vi "HFRR ADV v025 new software.vi"() -> ()   [LabVIEW 2025] (continued)
    shift-left: w3 -> [w1664]
    shift-right: [w1669] -> _
    shift-left: w3 -> [w1663]
    shift-right: [w1668] -> _
    shift-left: w3 -> [w1662]
    shift-right: [w1667] -> _
    shift-left: w3 -> [w1661]
    shift-right: [w1666] -> _
    shift-left: w3 -> [w1660]
    shift-right: [w1665] -> _
    shift-left: w3 -> [w1659]
    shift-right: [w1650] -> _
    shift-left: w3 -> [w1653]
    shift-right: [w1649] -> _
    shift-left: w3 -> [w1652]
    shift-right: [w1648] -> _
    shift-left: w3 -> [w1651]
    stop <- w1698 stop-if-true
    n1472 = local read "Read UNO"() -> (w1657:string)
    n1473 = local read "Error  2"() -> (w1697:errorcluster)
    n1474 = String Length(string=w1657) -> (length=w1656:i32)
    n1475 = call <vilib>:"Trim Whitespace.vi"("string"=w1657) -> ("trimmed string"=w1658:string)  [unwired: 1 in]
    n1476 = Greater Or Equal?(x=w1656, y=23) -> (x >= y?=w1654:bool)
    n1477 = case shown="No Error" w1697 {
      tunnel: w1696 -> [w1744 w1840]
      tunnel: w1695 -> [w1743 w1839]
      tunnel: w1694 -> [w1742 w1838]
      tunnel: w1693 -> [w1741 w1837]
      tunnel: [w1740 w1840] -> w1692
      tunnel: [w1739 w1839] -> w1691
      tunnel: [w1738 w1838] -> w1690
      tunnel: [w1737 w1837] -> w1689
      tunnel: w1688 -> [w1736 w1836]
      tunnel: [w1735 w1836] -> w1687
      tunnel: w1685 -> [w1734 w1835]
      tunnel: w1686 -> [w1733 w1834]
      tunnel: [w1732 w1835] -> w1684
      tunnel: [w1731 w1834] -> w1683
      tunnel: w1682 -> [w1730 w1833]
      tunnel: w1681 -> [w1729 w1832]
      tunnel: w1680 -> [w1728 w1831]
      tunnel: w1679 -> [w1727 w1830]
      tunnel: w1678 -> [w1726 w1829]
      tunnel: w1677 -> [w1725 w1828]
      tunnel: [w1724 w1833] -> w1676
      tunnel: [w1723 w1832] -> w1675
      tunnel: [w1722 w1831] -> w1674
      tunnel: [w1721 w1830] -> w1673
      tunnel: [w1720 w1829] -> w1672
      tunnel: [w1719 w1828] -> w1671
      tunnel: w1664 -> [w1718 w1827]
      tunnel: [w1717 w1827] -> w1670
      tunnel: [w1716 w1823] -> w1669
      tunnel: [w1715 w1822] -> w1668
      tunnel: [w1714 w1826] -> w1667
      tunnel: [w1713 w1825] -> w1666
      tunnel: [w1712 w1824] -> w1665
      tunnel: w1663 -> [w1711 w1826]
      tunnel: w1662 -> [w1710 w1825]
      tunnel: w1661 -> [w1709 w1824]
      tunnel: w1660 -> [w1708 w1823]
      tunnel: w1659 -> [w1707 w1822]
      tunnel: w1658 -> [w1706 _]
      tunnel: w1654 -> [w1705 _]
      tunnel: w1653 -> [w1704 w1821]
      tunnel: w1652 -> [w1703 w1820]
      tunnel: w1651 -> [w1702 w1819]
      tunnel: [w1701 w1821] -> w1650
      tunnel: [w1700 w1820] -> w1649
      tunnel: [w1699 w1819] -> w1648
      frame No Error {
        n1478 = case shown="True" w1705 {
          tunnel: w1744 -> [w1760 w1812]
          tunnel: w1743 -> [w1759 w1811]
          tunnel: w1742 -> [w1758 w1810]
          tunnel: w1741 -> [w1757 w1809]
          tunnel: [w1760 w1808] -> w1740
          tunnel: [w1759 w1807] -> w1739
          tunnel: [w1758 w1806] -> w1738
          tunnel: [w1757 w1805] -> w1737
          tunnel: w1736 -> [w1756 w1803]
          tunnel: [w1756 w1802] -> w1735
          tunnel: w1734 -> [w1755 w1801]
          tunnel: w1733 -> [w1754 w1800]
          tunnel: [w1755 w1799] -> w1732
          tunnel: [w1754 w1798] -> w1731
          tunnel: w1730 -> [w1753 w1797]
          tunnel: w1729 -> [w1752 w1796]
          tunnel: w1728 -> [w1751 w1795]
          tunnel: w1727 -> [w1750 w1794]
          tunnel: w1726 -> [w1749 w1793]
          tunnel: w1725 -> [w1748 w1792]
          tunnel: [w1753 w1791] -> w1724
          tunnel: [w1752 w1790] -> w1723
          tunnel: [w1751 w1789] -> w1722
          tunnel: [w1750 w1788] -> w1721
          tunnel: [w1749 w1787] -> w1720
          tunnel: [w1748 w1786] -> w1719
          tunnel: w1718 -> [w1766 w1785]
          tunnel: [w1766 w1784] -> w1717
          tunnel: [w1763 w1783] -> w1716
          tunnel: [w1762 w1782] -> w1715
          tunnel: [w1765 w1781] -> w1714
          tunnel: [w1761 w1780] -> w1713
          tunnel: [w1764 w1779] -> w1712
          tunnel: w1711 -> [w1765 w1778]
          tunnel: w1710 -> [w1764 w1777]
          tunnel: w1709 -> [w1763 w1776]
          tunnel: w1708 -> [w1762 w1775]
          tunnel: w1707 -> [w1761 w1774]
          tunnel: w1706 -> [_ w1773]
          tunnel: w1704 -> [w1747 w1772]
          tunnel: w1703 -> [w1746 w1771]
          tunnel: w1702 -> [w1745 w1770]
          tunnel: [w1747 w1769] -> w1701
          tunnel: [w1746 w1768] -> w1700
          tunnel: [w1745 w1767] -> w1699
          frame False {
          }
          frame True {
            n1479 = Tick Count (ms)() -> (millisecond timer value=w1804:u32)
            n1480 = String To Byte Array(string=w1773) -> (unsigned byte array=w1817:u8[])
            n1481 = Array Size(array=w1817) -> (size(s)=w1816:i32)
            n1482 = formula code="// --- INTERNAL VARIABLE DECLARATIONS ---\nint i = 0;\nint k = 0;\nint start_idx = -1;\nint end_idx = -1;\nint phase = 0;\nint sign0 = 1;\nint sign1 = 1;\nint ch0_val = 0;   \nint ch1_val = 0;   \nfloat ch0_raw = 0.0;\nfloat ch1_raw = 0.0;\nfloat temp0 = 0.0;\nfloat temp1 = 0.0;\nfloat ch0_clean = 0.0;\nfloat ch1_clean = 0.0;\n\n// Temporal intermediate variables for calculation smoothing\nfloat raw_p2p_v = 0.0;\nfloat raw_friction = 0.0;\nfloat raw_cof = 0.0;\n\n// Initialize output variables to current shift register states right away\nout_LVDT_Min_V = in_LVDT_Min_V;\nout_LVDT_Max_V = in_LVDT_Max_V;\nout_LVDT_P2P_V = in_LVDT_P2P_V;\nout_Piezo_P2P = in_Piezo_P2P;\nout_Friction_N = in_Friction_N;\nout_COF = in_COF;\nwindow_ready = 0;\n\n// --- STEP 1: PARSE EVERY STRING IN THE BYTE ARRAY ---\nif (array_size > 2) {\n    for (i = 0; i < array_size - 1; i++) {\n        if (raw_bytes[i] == 42) { // '*' character detected\n            start_idx = i;\n        }\n        \n        // Match standard delimiter sequence \";&\" or end window character\n        if (raw_bytes[i] == 59 && raw_bytes[i+1] == 38 && start_idx != -1) { \n            end_idx = i;\n            ch0_val = 0;\n            ch1_val = 0;\n            sign0 = 1;\n            sign1 = 1;\n            phase = 0; \n\n            for (k = start_idx + 1; k < end_idx; k++) {\n                if (raw_bytes[k] == 45) { // '-' sign\n                    if (phase == 0) sign0 = -1;\n                    else sign1 = -1;\n                }\n                else if (raw_bytes[k] == 43) { // '+' sign\n                    if (phase == 0) sign0 = 1;\n                    else sign1 = 1;\n                }\n                else if (raw_bytes[k] == 59) { // ';' delimiter\n                    phase = 1; \n                }\n                else if (raw_bytes[k] >= 48 && raw_bytes[k] <= 57) { // Numeric ASCII digits\n                    if (phase == 0) {\n                        ch0_val = (ch0_val * 10) + (raw_bytes[k] - 48);\n                    } else {\n                        ch1_val = (ch1_val * 10) + (raw_bytes[k] - 48);\n                    }\n                }\n            }\n\n            // Implicit type conversion\n            ch0_raw = ch0_val * sign0 * 1.0;\n            ch1_raw = ch1_val * sign1 * 1.0;\n\n            // --- STEP 2: 3-SAMPLE MEDIAN FILTER ---\n            m0_2 = m0_1; m0_1 = m0_0; m0_0 = ch0_raw;\n            float s0_0 = m0_0; float s0_1 = m0_1; float s0_2 = m0_2;\n            if (s0_0 > s0_1) { temp0 = s0_0; s0_0 = s0_1; s0_1 = temp0; }\n            if (s0_1 > s0_2) { temp0 = s0_1; s0_1 = s0_2; s0_2 = temp0; }\n            if (s0_0 > s0_1) { temp0 = s0_0; s0_0 = s0_1; s0_1 = temp0; }\n            ch0_clean = s0_1;\n\n            m1_2 = m1_1; m1_1 = m1_0; m1_0 = ch1_raw;\n            float s1_0 = m1_0; float s1_1 = m1_1; float s1_2 = m1_2;\n            if (s1_0 > s1_1) { temp1 = s1_0; s1_0 = s1_1; s1_1 = temp1; }\n            if (s1_1 > s1_2) { temp1 = s1_1; s1_1 = s1_2; s1_2 = temp1; }\n            if (s1_0 > s1_1) { temp1 = s1_0; s1_0 = s1_1; s1_1 = temp1; }\n            ch1_clean = s1_1;\n\n            // --- STEP 3: EXPONENTIAL FILTER (STREAM LEVEL) ---\n            if (ch0_filt == 0.0) ch0_filt = ch0_clean;\n            if (ch1_filt == 0.0) ch1_filt = ch1_clean;\n\n            ch0_filt = ch0_filt + (ch0_clean - ch0_filt) * 0.125;\n            ch1_filt = ch1_filt + (ch1_clean - ch1_filt) * 0.125;\n\n            // --- STEP 4: MIN/MAX WINDOW CONTINUOUS ACCUMULATION ---\n            if (ch0_filt > max_ch0) max_ch0 = ch0_filt;\n            if (ch0_filt < min_ch0) min_ch0 = ch0_filt;\n            if (ch1_filt > max_ch1) max_ch1 = ch1_filt;\n            if (ch1_filt < min_ch1) min_ch1 = ch1_filt;\n\n            start_idx = -1; \n        }\n    }\n}\n\n// --- STEP 5: WINDOW EVALUATION ENGINE ---\nif (((current_time_ms - start_time_ms) >= 50) && (min_ch0 < 9000000.0) && (max_ch0 > -9000000.0)) {\n    window_ready = 1;\n\n    // Linear Bit-to-Voltage Transformations\n    out_LVDT_Min_V = (min_ch0 * VREF) / 8388607.0;\n    out_LVDT_Max_V = (max_ch0 * VREF) / 8388607.0;\n    raw_p2p_v = out_LVDT_Max_V - out_LVDT_Min_V;\n\n    // Piezo scaling calculations\n    out_Piezo_P2P = max_ch1 - min_ch1;\n    raw_friction = out_Piezo_P2P * PIEZO_CAL_FACTOR;\n    raw_cof = raw_friction / NORMAL_FORCE;\n\n    // --- STEP 6: OUTPUT METRIC SMOOTHING (Low-Pass Filter Alpha = 0.20) ---\n    // Seed initial historical metrics if first loop iteration\n    if (hist_LVDT_P2P == 0.0) hist_LVDT_P2P = raw_p2p_v;\n    if (hist_Friction == 0.0) hist_Friction = raw_friction;\n    if (hist_COF == 0.0)      hist_COF = raw_cof;\n\n    // Apply exponential output dampening\n    hist_LVDT_P2P = hist_LVDT_P2P + (raw_p2p_v - hist_LVDT_P2P) * 0.05;\n    hist_Friction = hist_Friction + (raw_friction - hist_Friction) * 0.05;\n    hist_COF      = hist_COF + (raw_cof - hist_COF) * 0.05;\n\n    // Direct smoothed parameters out to UI Indicators\n    out_LVDT_P2P_V = hist_LVDT_P2P;\n    out_Friction_N = hist_Friction;\n    out_COF        = hist_COF;\n\n    // Reset tracking targets to extreme boundaries safely\n    min_ch0 = 9999999.0;\n    max_ch0 = -9999999.0;\n    min_ch1 = 9999999.0;\n    max_ch1 = -9999999.0;\n\n    start_time_ms = current_time_ms;\n}"("raw_bytes"=w1817, "array_size"=w1816, "VREF"="VREF", "PIEZO_CAL_FACTOR"="PIEZO_CAL_FACTOR", "NORMAL_FORCE"="NORMAL_FORCE", "min_ch0"=w1812, "max_ch0"=w1811, "min_ch1"=w1810, "max_ch1"=w1809, "current_time_ms"=w1804, "start_time_ms"=w1803, "ch0_filt"=w1801, "ch1_filt"=w1800, "m0_0"=w1797, "m0_1"=w1796, "m0_2"=w1795, "m1_0"=w1794, "m1_1"=w1793, "m1_2"=w1792, "in_LVDT_Min_V"=w1785, "in_LVDT_Max_V"=w1778, "in_LVDT_P2P_V"=w1777, "in_Piezo_P2P"=w1776, "in_Friction_N"=w1775, "in_COF"=w1774, "hist_LVDT_P2P"=w1772, "hist_Friction"=w1771, "hist_COF"=w1770) -> ("window_ready"=→"Valid_data":dbl, "out_LVDT_Min_V"=w1784:dbl, "out_LVDT_Max_V"=w1783:dbl, "out_LVDT_P2P_V"=w1782:dbl, "out_Piezo_P2P"=w1781:dbl, "out_Friction_N"=w1780:dbl, "out_COF"=w1779:dbl, "min_ch0"=w1808:dbl, "max_ch0"=w1807:dbl, "min_ch1"=w1806:dbl, "max_ch1"=w1805:dbl, "start_time_ms"=w1802:u32, "ch0_filt"=w1799:dbl, "ch1_filt"=w1798:dbl, "m0_0"=w1791:dbl, "m0_1"=w1790:dbl, "m0_2"=w1789:dbl, "m1_0"=w1788:dbl, "m1_1"=w1787:dbl, "m1_2"=w1786:dbl, "hist_LVDT_P2P"=w1769:dbl, "hist_Friction"=w1768:dbl, "hist_COF"=w1767:dbl)
            "LVDT MIN" <- w1784
            "LVDT MAX" <- w1783
            "LVDT Peak" <- w1782
            "pizo raw" <- w1781
            "Friction" <- w1780
            "cof" <- w1779
          }
        }
      }
      frame Error {
      }
    }
    n1483 = local read "Quit"() -> (w1698:bool)
  }
  n1484 = disable-structure shown="Disabled" {
    disable-tunnel: errorcluster {"status"=TRUE, "code"=0, "source"="Init"} ("error IO") -> [w1843 _]
    disable-tunnel: [w1841 _] -> w46
    frame Disabled {
      n1485 = while {
        shift-right: [w1859] -> w1845
        shift-left: _ -> [w1850]
        shift-right: [w1858] -> w1844
        shift-left: w1843 -> [w1852]
        tunnel: [w1847] -> w1841
        tunnel: [w1857] -> _
        i -> [w1857]
        stop <- w1847 stop-if-true
        n1486 = local read "Port 1a"() -> (w1853:bool)
        n1487 = local read "Port 3"() -> (w1854:bool)
        n1488 = local read "Com Port 1"() -> (w1851:refnum<visa-resource-name>)
        n1489 = Or(x=w1854, y=w1853) -> (x .or. y?=w1856:bool)
        n1490 = Unbundle(w1852) -> ("status"=→"Port 3":bool)  [unwired: 2 out]
        n1491 = Not Equal?(x=w1851, y=w1850) -> (x != y?=w1848:bool)
        n1492 = case shown="True" w1856 {
          frame False {
            w1862 = TRUE ("Visible")
            n1493 = property on="Port 1a" class="Bool (strict)"("Visible"=w1862) -> ()  [unwired: 2 in, 2 out]
            n1494 = property on="Port 3" class="Bool (strict)"("Visible"=w1862) -> ()  [unwired: 2 in, 2 out]
          }
          frame True {
            w1863 = TRUE ("Visible")
            n1495 = property on="Port 1a" class="Bool (strict)"("Visible"=w1863) -> ()  [unwired: 2 in, 2 out]
            n1496 = property on="Port 3" class="Bool (strict)"("Visible"=w1863) -> ()  [unwired: 2 in, 2 out]
          }
        }
        n1497 = Wait (ms)(milliseconds to wait=u32 40) -> ()  [unwired: 1 out]
        n1498 = case shown="True" w1848 {
          tunnel: [w1860 errorcluster {"status"=TRUE, "code"=0, "source"="Init"} ("error out")] -> w1849
          tunnel: w1852 -> [w1860 _]
          frame False {
          }
          frame True {
          }
        }
        n1499 = case shown="Error" w1849 {
          selector: w1849 -> [w1870 w1888]
          tunnel: [w1873 w1892] -> w1859
          tunnel: [w1872 w1886] -> w1858
          tunnel: w1850 -> [w1871 w1890]
          frame No Error {
            n1500 = property class="Instr"(reference=w1871, error in=w1870) -> (reference out=w1868:refnum<visa-resource-name>, error out=w1869:errorcluster, "Serial Settings:Number of Bytes at Serial Port"=w1865:u32)
            n1501 = Greater?(x=w1865, y=u32 5) -> (0:w1864:bool)
            n1502 = Not(x=w1864) -> (.not. x?=→"Port 1a":bool)
            n1503 = while {
              tunnel: [w1881] -> w1872
              tunnel: [w1880] -> w1873
              tunnel: w1869 -> [w1879]
              tunnel: w1868 -> [w1878]
              stop <- TRUE stop-if-true
              n1504 = property class="Instr" props=["Serial Settings:Number of Bytes at Serial Port"](reference=w1878, error in=w1879) -> (reference out=w1883:refnum<visa-resource-name>, error out=w1882:errorcluster)  [unwired: 1 out]
              n1505 = VISA Read(VISA resource name=w1883, byte count=u32 50, error in (no error)=w1882) -> (VISA resource name out=w1880:refnum<visa-resource-name>, read buffer=w1875:string, error out=w1881:errorcluster)  [unwired: 1 out]
              n1506 = Wait (ms)(milliseconds to wait=u32 5) -> ()  [unwired: 1 out]
            }
          }
          frame Error {
            w1898 = u16 0 items=["None", "XON/XOFF", "RTS/CTS", "XON/XOFF & RTS/CTS", "DTR/DSR", "XON/XOFF & DTR/DSR"] ("flow control (0:none)  2")
            w1896 = u16 10 items=["1.0"=10, "1.5"=15, "2.0"=20] ("stop bits 2")
            w1894 = u16 0 items=["None", "Odd", "Even", "Mark", "Space"] ("parity 2")
            w1895 = u32 10000  # timeout (10sec)
            n1507 = VISA Close(VISA resource name=w1890, error in (no error)=w1888) -> (error out=w1891:errorcluster)
            n1508 = local write "Port 1a"(FALSE ("Port 1a")) -> ()
            n1509 = local read "Com Port 1"() -> (w1885:refnum<visa-resource-name>)
            n1510 = call <vilib>:"Clear Errors.vi"("error in (no error)"=w1891) -> ("error out"=w1889:errorcluster)  [unwired: 5 in, 1 out]
            n1511 = call-poly "VISA Configure Serial Port"("VISA resource name"=w1885, "timeout (10sec)"=w1895, "baud rate (9600)"=u32 250000 ("baud rate  2"), "data bits (8)"=u16 8 ("data bits  2"), "parity (0:none)"=w1894, "error in (no error)"=w1889, "stop bits (10: 1 bit)"=w1896, "flow control (0:none)"=w1898) -> ("VISA resource name out"=w1899:refnum<visa-resource-name>, "error out"=w1900:errorcluster)  [unwired: 6 in]
            n1512 = flat-sequence {
              tunnel: w1899 -> [w1902]
              tunnel: w1900 -> [w1901]
              tunnel: [w1902] -> w1892
              tunnel: [w1901] -> w1886
              frame #0 {
                n1513 = Wait (ms)(milliseconds to wait=u32 50) -> ()  [unwired: 1 out]
              }
            }
            "Residual Uno" <- ""
          }
        }
        n1514 = local read "Quit"() -> (w1847:bool)
        "Error Uno" <- w1852
      }
      n1515 = VISA Close(VISA resource name=w1845, error in (no error)=w1844) -> (error out=w1842:errorcluster)
      n1516 = call <vilib>:"Clear Errors.vi"("error in (no error)"=w1842) -> ()  [unwired: 5 in, 2 out]
    }
    frame Enabled {
    }
  }
  n1517 = while {
    stop <- w1913 stop-if-true
    # "V0OLTAGE TO STROKE (peice vise calibration)"
    n1518 = local read "LVDT MIN"() -> (w1905:dbl)
    n1519 = local read "LVDT Peak"() -> (w1904:dbl)
    n1520 = Wait (ms)(milliseconds to wait=u32 10) -> ()  [unwired: 1 out]
    n1521 = formula code="// Dynamic Parameterized Linear Interpolation Node\n// Inputs: vpp_val, voltages (Array), distances (Array)\n// Outputs: stroke\n\nint i = 0;\nint segments = 11; // 12 points make 11 interpolation segments\n\n// 1. Lower Boundary Clamp\nif (vpp_val <= voltages[0]) {\n    stroke = distances[0];\n}\n// 2. Upper Boundary Clamp\nelse if (vpp_val >= voltages[segments]) {\n    stroke = distances[segments];\n}\n// 3. Dynamic Segment Search Loop\nelse {\n    stroke = distances[0]; // Fallback baseline\n    for (i = 0; i < segments; i++) {\n        if (vpp_val >= voltages[i] && vpp_val <= voltages[i+1]) {\n            // Standard linear interpolation formula using array lookups\n            stroke = distances[i] + (vpp_val - voltages[i]) * (distances[i+1] - distances[i]) / (voltages[i+1] - voltages[i]);\n            break; // Segment found, safely exit the loop\n        }\n    }\n}"("vpp_val"=w1904, "voltages"="calibration values", "distances"="STROKE") -> ("stroke"=→"LVDT STROKE":dbl)
    n1522 = local read "Calibration Tare Value"() -> (w1909:dbl)
    n1523 = local read "Calibration Tare"() -> (w1907:bool)
    n1524 = Subtract(x=w1905, y=w1909) -> (x-y=→"LVDT STROKE  Calibration":dbl)
    n1525 = case shown="True" w1907 {
      selector: w1907 -> [_ w1915]
      tunnel: w1905 -> [_ w1916]
      frame False {
      }
      frame True {
        n1526 = Not(x=w1915) -> (.not. x?=w1914:bool)
        n1527 = local write "Calibration Tare"(w1914) -> ()
        "Calibration Tare Value" <- w1916
      }
    }
    n1528 = local read "Quit"() -> (w1913:bool)
  }
  n1529 = while {
    stop <- w1936 stop-if-true
    n1530 = call <vilib>:"High Resolution Polling Wait.vi"("seconds to wait"=0.02) -> ()  [unwired: 10 in, 1 out]
    n1531 = local read "Due read"() -> (w1934:string)
    n1532 = Spreadsheet String To Array(delimiter (Tab)=";", format string="", spreadsheet string=w1934, array type (2D Dbl)=string[] []) -> (array=w1931:string[])
    n1533 = Fract/Exp String To Number(string=w1931) -> (number=w1930:dbl[])  [unwired: 3 in, 1 out]
    n1534 = Index Array(array=w1930) -> (element #1=→"Sample Temperature":dbl, element #2=→"Target Sample Temperature":dbl, element #3=→"Current Duty Cycle":dbl, element #4=→"Ambient Temperature":dbl, element #5=→"Dac Status":dbl, element #6=→"Vpp":dbl, element #7=→"Active Error Code":dbl, element #8=→"Kp":dbl, element #9=→"Ki":dbl, element #10=→"Kd":dbl, element #11=→"SampleRaw":dbl, element #12=→"AmbRaw":dbl)  [unwired: 12 in]
    n1535 = local read "Quit"() -> (w1936:bool)
  }
  n1536 = while {
    shift-right: [w1950] -> w41
    shift-left: _ -> [w1942]
    shift-right: [w1937] -> w40
    shift-left: errorcluster {"status"=FALSE, "code"=0, "source"="Init"} ("error out") -> [w1944]
    tunnel: [w1939] -> w45
    tunnel: [w1949] -> _
    i -> [w1949]
    stop <- w1939 stop-if-true
    n1537 = local read "Com Port 2"() -> (w1943:refnum<visa-resource-name>)
    n1538 = local read "Port 2a"() -> (w1945:bool)
    n1539 = Unbundle(w1944) -> ("status"=→"Port 4":bool)  [unwired: 2 out]
    n1540 = call <vilib>:"High Resolution Polling Wait.vi"("seconds to wait"=0.02) -> ()  [unwired: 10 in, 1 out]
    n1541 = local read "Port 4"() -> (w1946:bool)
    n1542 = Not Equal?(x=w1943, y=w1942) -> (x != y?=w1941:bool)
    n1543 = Or(x=w1946, y=w1945) -> (x .or. y?=w1948:bool)
    n1544 = case shown="False" w1948 {
      frame False {
        w1953 = TRUE ("Visible")
        n1545 = property on="Port 2a" class="Bool (strict)"("Visible"=w1953) -> ()  [unwired: 2 in, 2 out]
        n1546 = property on="Port 4" class="Bool (strict)"("Visible"=w1953) -> ()  [unwired: 2 in, 2 out]
      }
      frame True {
        w1954 = TRUE ("Visible")
        n1547 = property on="Port 2a" class="Bool (strict)"("Visible"=w1954) -> ()  [unwired: 2 in, 2 out]
        n1548 = property on="Port 4" class="Bool (strict)"("Visible"=w1954) -> ()  [unwired: 2 in, 2 out]
      }
    }
    n1549 = case shown="True" w1941 {
      tunnel: [w1951 errorcluster {"status"=TRUE, "code"=0, "source"="Init"} ("error out")] -> w1940
      tunnel: w1944 -> [w1951 _]
      frame False {
      }
      frame True {
      }
    }
    n1550 = case shown="No Error" w1940 {
      selector: w1940 -> [w1967 w1998]
      tunnel: [w1960 w2003] -> w1950
      tunnel: [w1968 w1996] -> w1937
      tunnel: w1942 -> [w1969 w2001]
      frame No Error {
        n1551 = property class="Instr" props=["Serial Settings:Number of Bytes at Serial Port"](reference=w1969, error in=w1967) -> (reference out=w1961:refnum<visa-resource-name>, error out=w1966:errorcluster)  [unwired: 1 out]
        n1552 = while {
          tunnel: [w1977] -> w1962
          tunnel: [w1976] -> w1963
          tunnel: w1966 -> [w1975]
          tunnel: w1961 -> [w1974]
          tunnel: [w1973] -> _
          i -> [w1973]
          stop <- TRUE stop-if-true
          n1553 = property class="Instr" props=["Serial Settings:Number of Bytes at Serial Port"](reference=w1974, error in=w1975) -> (reference out=w1979:refnum<visa-resource-name>, error out=w1978:errorcluster)  [unwired: 1 out]
          n1554 = VISA Read(VISA resource name=w1979, byte count=u32 1000, error in (no error)=w1978) -> (VISA resource name out=w1976:refnum<visa-resource-name>, read buffer=→"Due read":string, error out=w1977:errorcluster)  [unwired: 1 out]
        }
        n1555 = local read "Due Write"() -> (w1959:string)
        n1556 = call <vilib>:"Trim Whitespace.vi"("string"=w1959) -> ("trimmed string"=w1958:string)  [unwired: 1 in]
        n1557 = Not Equal?(x=w1958, y="") -> (x != y?=w1964:bool)
        n1558 = VISA Flush I/O Buffer(VISA resource name=w1963) -> (VISA resource name out=w1956:refnum<visa-resource-name>, error out=→"error out 10":errorcluster)  [unwired: 2 in]
        n1559 = case shown="True" w1964 {
          tunnel: w1956 -> [w1981 w1986]
          tunnel: [w1981 w1990] -> w1960
          tunnel: w1962 -> [w1980 w1985]
          tunnel: [w1980 w1988] -> w1968
          tunnel: w1958 -> [_ w1984]
          tunnel: [_ w1987] -> _
          frame False {
            # "DATA  WRITE LOOP"
          }
          frame True {
            n1560 = Concatenate Strings(w1984, "\r\n") -> (w1983:string)
            n1561 = VISA Write(VISA resource name=w1986, write buffer=w1983, error in (no error)=w1985) -> (VISA resource name out=w1990:refnum<visa-resource-name>, return count=w1987:u32, error out=w1989:errorcluster)
            n1562 = flat-sequence {
              tunnel: w1989 -> [w1992]
              tunnel: [w1992] -> w1988
              frame #0 {
                n1563 = local write "Due Write"("" ("Command")) -> ()
                n1564 = Wait (ms)(milliseconds to wait=u32 5) -> ()  [unwired: 1 out]
              }
            }
          }
        }
        "Port 2a" <- TRUE ("Port 2a")
      }
      frame Error {
        w2009 = u16 0 items=["None", "XON/XOFF", "RTS/CTS", "XON/XOFF & RTS/CTS", "DTR/DSR", "XON/XOFF & DTR/DSR"] ("flow control (0:none)  2")
        w2007 = u16 10 items=["1.0"=10, "1.5"=15, "2.0"=20] ("stop bits 2")
        w2005 = u16 0 items=["None", "Odd", "Even", "Mark", "Space"] ("parity 2")
        w2006 = u32 10000  # timeout (10sec)
        n1565 = VISA Clear(VISA resource name=w2001, error in (no error)=w1998) -> (VISA resource name out=w2000:refnum<visa-resource-name>, error out=w1999:errorcluster)
        n1566 = VISA Close(VISA resource name=w2000, error in (no error)=w1999) -> (error out=w2002:errorcluster)
        n1567 = call <vilib>:"Clear Errors.vi"("error in (no error)"=w2002) -> ()  [unwired: 5 in, 2 out]
        n1568 = local write "Port 2a"(FALSE ("Port 2a")) -> ()
        n1569 = local read "Com Port 2"() -> (w1995:refnum<visa-resource-name>)
        "visa due" <- w1995
        n1570 = call-poly "VISA Configure Serial Port"("VISA resource name"=w1995, "timeout (10sec)"=w2006, "baud rate (9600)"=u32 250000 ("baud rate  2"), "data bits (8)"=u16 8 ("data bits  2"), "parity (0:none)"=w2005, "stop bits (10: 1 bit)"=w2007, "flow control (0:none)"=w2009) -> ("VISA resource name out"=w2010:refnum<visa-resource-name>, "error out"=w2011:errorcluster)  [unwired: 7 in]
        n1571 = flat-sequence {
          tunnel: w2010 -> [w2013]
          tunnel: w2011 -> [w2012]
          tunnel: [w2013] -> w2003
          tunnel: [w2012] -> w1996
          frame #0 {
            n1572 = Wait (ms)(milliseconds to wait=u32 50) -> ()  [unwired: 1 out]
          }
        }
        "Residual Due" <- ""
      }
    }
    "error out 9" <- w1937
    n1573 = local read "Quit"() -> (w1939:bool)
    "Error Due" <- w1944
  }
  n1574 = local write "FRICVALZ"(0.0 ("FRICVALZ")) -> ()
  n1575 = property on="RUN" class="Bool (strict)"("Visible"=TRUE) -> ()  [unwired: 2 in, 2 out]
  n1576 = while {
    tunnel: [w2028] -> _
    tunnel: [w2015] -> w55
    i -> [w2028]
    stop <- w2015 stop-if-true
    n1577 = local read "conststatus"() -> (w2019:dbl)
    n1578 = local read "Main Tab"() -> (w2017:T2)
    n1579 = local read "EDIT"() -> (w2034:bool)
    n1580 = local read "Rate"() -> (w2033:dbl)
    n1581 = case shown="True" w2034 {
      tunnel: [FALSE TRUE] -> _
      frame False {
      }
      frame True {
      }
    }
    n1582 = Equal?(x=w2017, y=T25."About" ("Main Tab")) -> (x = y?=w2026:bool)
    n1583 = Equal?(x=w2019, y=0.0) -> (x = y?=w2020:bool)
    n1584 = Divide(x=1.0, y=w2033) -> (x/y=w2029:dbl)
    "Time 2" <- w2029
    n1585 = case shown="True" w2020 {
      frame False {
      }
      frame True {
        # "C:\\WinDucom\\calibrate WO 2391.dcf"
        n1586 = local write "Lan flag"(22) -> ()
        n1587 = local write "conststatus"(10.0 ("rpm value : 2")) -> ()
        n1588 = String To Path(string="C:\\LAB-IQ\\calibrate WO 2465.dcf") -> (path=w2040:path)
        n1589 = Open/Create/Replace File "Open File"(file path (use dialog)=w2040) -> (refnum out=w2038:refnum<file>)  [unwired: 5 in, 2 out]
        n1590 = for {
          N: 23 -> [_]
          tunnel: w2038 -> [w2049]
          i -> [w2043]
          (unwired) TRUE ("line mode (F)")
          n1591 = Read from Text File "Read File"(file (use dialog)=w2049) -> (text=w2048:string)  [unwired: 3 in, 3 out]
          n1592 = Match Pattern(string=w2048, regular expression="]") -> (after substring=w2046:string)  [unwired: 1 in, 3 out]
          n1593 = String Subset(string=w2048, offset (0)=5, length (rest)=10 ("length (rest)")) -> (substring=w2041:string)
          n1594 = Fract/Exp String To Number(string=w2041) -> (number=w2042:dbl)  [unwired: 3 in, 1 out]
          n1595 = Match Pattern(string=w2046, regular expression="-") -> (before substring=w2044:string)  [unwired: 1 in, 3 out]
          n1596 = case shown="18" w2043 {
            tunnel: w2042 -> [_ _ _ _ _ _ _ _ _ _ w2056 _ _ _ _ _ _ _ _ _ _ _ _ _]
            tunnel: w2044 -> [_ _ _ _ w2052 w2053 w2054 _ _ _ _ _ _ _ _ _ _ _ _ _ w2057 w2058 w2059 _]
            frame 0 {
            }
            frame 1 {
            }
            frame 2 {
            }
            frame 3 {
            }
            frame 4 {
              n1597 = local write "Com Port 1"(w2052) -> ()
            }
            frame 5 {
              n1598 = local write "Com Port 2"(w2053) -> ()
              n1599 = local write "visa due"(w2053) -> ()
            }
            frame 6 {
              n1600 = String To Path(string=w2054) -> (path=w2055:path)
              n1601 = local write "File Path"(w2055) -> ()
              "String" <- w2054
            }
            frame 7 {
            }
            frame 8 {
            }
            frame 9 {
            }
            frame 10 {
              n1602 = local write "Language Selection"(w2056) -> ()
            }
            frame 11 {
            }
            frame 12 {
            }
            frame 13 {
            }
            frame 14 {
            }
            frame 15 {
            }
            frame 16 {
            }
            frame 17 {
            }
            frame 18 {
            }
            frame 21 {
            }
            frame 22 {
              n1603 = local write "Com Port 3"(w2057) -> ()
            }
            frame 20 {
              n1604 = local write "Camera Port :"(w2058) -> ()
            }
            frame 19 {
              n1605 = local write "C3 :"(w2059) -> ()
            }
            frame 23, Default {
            }
          }
        }
      }
    }
    n1606 = Select(t=u32 2500 ("milliseconds to wait"), s=w2026, f=u32 500 ("milliseconds to wait")) -> (s? t:f=w2024:u32)
    n1607 = Multiply(x=w2029, y=w2024) -> (x*y=w2031:dbl)
    n1608 = call "Elapsed Time2"("Time Target (s)"=w2031, "Auto Reset"=TRUE) -> ("Time has Elapsed"=w2021:bool)  [unwired: 10 in, 7 out]
    n1609 = case shown="True" w2021 {
      frame False {
      }
      frame True {
        n1610 = stacked-sequence {
          frame #0 {
            # "DATA PROCESSING"
            # "115 mV/N"
            n1611 = local read "Sample Temperature"() -> (w2062:dbl)
            n1612 = local read "RH Numeric:"() -> (→"Humidity ( %RH )" →"Hum" →"Hum 2":dbl)
            n1613 = local read "FRICVALZ"() -> (w2079:dbl)
            n1614 = local read "Friction"() -> (w2065:dbl)
            n1615 = call <vilib>:"Mean PtByPt.vi"("x"=w2062, "sample length"=100) -> ("mean"=w2061:dbl)  [unwired: 2 in, 1 out]
            "TEMP 2" <- w2061
            "TEMP 3" <- w2061
            n1616 = Subtract(x=w2065, y=w2079) -> (x-y=w2074:dbl)
            "FF 2" <- w2074
            "FF 4" <- w2074
            n1617 = local read "Ambient Temperature"() -> (→"AIR TEMP":dbl)
            n1618 = local read "TEMP"() -> (w2078:dbl)
            n1619 = local write "FF 3"(w2074) -> ()
            n1620 = Compound Arithmetic op=OR("FRICVALZ 4", "FRICVALZ 3", "FRICVALZ 2") -> (w2070:bool)
            n1621 = case shown="True" w2070 {
              tunnel: w2065 -> [_ w2085]
              frame False {
              }
              frame True {
                w2084 = FALSE ("FRICVALZ")
                n1622 = local write "FRICVALZ 3"(w2084) -> ()
                n1623 = local write "FRICVALZ 2"(w2084) -> ()
                n1624 = local write "FRICVALZ 4"(w2084) -> ()
                "FRICVALZ" <- w2085
              }
            }
            n1625 = Not A Number/Path/Refnum?(number/path/refnum=w2078) -> (NaN/Path/Refnum?=w2077:bool)
            n1626 = Not A Number/Path/Refnum?(number/path/refnum=w2074) -> (NaN/Path/Refnum?=w2076:bool)
            n1627 = Divide(x=w2074, y=1.96) -> (x/y=w2071:dbl)
            n1628 = Compound Arithmetic op=OR(w2077, w2076) -> (w2075:bool)
            n1629 = Not A Number/Path/Refnum?(number/path/refnum=w2071) -> (NaN/Path/Refnum?=w2072:bool)
            n1630 = case shown="True" w2075 {
              frame False {
              }
              frame True {
                n1631 = local write "TEMP"(0.0 ("TEMP")) -> ()
                n1632 = local write "FF 2"(0.0 ("FF 2")) -> ()
                n1633 = local write "reinit"(TRUE ("reinit")) -> ()
              }
            }
            n1634 = local write "TEMP"(w2061) -> ()
            n1635 = Select(t=0.0, s=w2072, f=w2071) -> (s? t:f=w2064:dbl)
            "COF 2" <- w2064
            n1636 = local write "COF 3"(w2064) -> ()
          }
        }
      }
    }
    n1637 = Wait (ms)(milliseconds to wait=u32 50) -> ()  [unwired: 1 out]
    n1638 = local read "Quit"() -> (w2015:bool)
    "Rate" <- 2500.0 ("No of Samples")
  }
  n1639 = while {
    tunnel: [w2112] -> _
    tunnel: [w2088] -> w57
    tunnel: w1 -> [_]
    i -> [w2112]
    stop <- w2088 stop-if-true
    # "C:\\LAB-IQ-NXT\\Scar View.exe"
    n1640 = local read "OK Button 16"() -> (w2101:bool)
    n1641 = local read "Main Tab"() -> (w2094:T2)
    n1642 = local read "service 3"() -> (w2095:bool)
    n1643 = local read "OPEN 6"() -> (w2097:bool)
    n1644 = local read "EDIT 2"() -> (w2099:bool)
    n1645 = flat-sequence {
      frame #0 {
        n1646 = stacked-sequence {
          frame #0 {
            n1647 = local read "EDIT"() -> (w2720:bool)
            n1648 = case shown="False" w2720 {
              tunnel: [u8 2 ("Disabled") u8 0 ("Disabled")] -> _
              frame False {
                w2722 = FALSE
                n1649 = local write "Password"("") -> ()
                n1650 = local write "x = y?"(w2722) -> ()
                n1651 = property on="Password" class="Str"("Visible"=w2722) -> ()  [unwired: 2 in, 2 out]
              }
              frame True {
                n1652 = property on="Password" class="Str"("Visible"=TRUE) -> ()  [unwired: 2 in, 2 out]
              }
            }
            "dipl pwd" <- "@143$\n" ("dipl pwd")
          }
          frame #1 {
          }
          frame #2 {
          }
          frame #3 {
          }
          frame #4 {
            n1653 = String To Byte Array(string="Password") -> (unsigned byte array=w2733:u8[])
            n1654 = Search 1D Array(1D array=w2733, element=u8 10) -> (index of element=w2731:i32)  [unwired: 1 in]
            n1655 = Index Array(array=w2733, index=w2731) -> (element=w2732:u8)
            n1656 = Equal?(x=w2732, y=10) -> (x = y?=w2728:bool)
            n1657 = case shown="True" w2728 {
              frame False {
              }
              frame True {
                # "password"
                # "password"
                n1658 = local read "Password"() -> (w2745:string)
                n1659 = String To Byte Array(string=w2745) -> (unsigned byte array=w2748:u8[])
                n1660 = String To Byte Array(string="@143$\n") -> (unsigned byte array=w2735:u8[])
                n1661 = Array Size(array=w2748) -> (size(s)=w2744:i32)
                n1662 = Array Size(array=w2735) -> (size(s)=w2740:i32)
                n1663 = for {
                  N: w2744 -> [_]
                  tunnel: w2748 -> [w2761]
                  tunnel: [w2759] -> w2749 mode=indexing
                  tunnel: w2744 -> [w2756]
                  i -> [w2757]
                  n1664 = Decrement(x=w2756) -> (x-1=w2755:i32)
                  n1665 = Index Array(array=w2761, index=w2757) -> (element=w2760:u8)
                  n1666 = Equal?(x=w2757, y=w2755) -> (x = y?=w2754:bool)
                  n1667 = Number To Decimal String(number=w2760) -> (decimal integer string=w2758:string)  [unwired: 1 in]
                  n1668 = Select(t="", s=w2754, f="\r") -> (s? t:f=w2751:string)
                  n1669 = Concatenate Strings(w2758, w2751) -> (w2759:string)
                }
                n1670 = for {
                  N: w2740 -> [_]
                  tunnel: w2735 -> [w2772]
                  tunnel: [w2770] -> w2738 mode=indexing
                  tunnel: w2740 -> [w2767]
                  i -> [w2768]
                  n1671 = Decrement(x=w2767) -> (x-1=w2766:i32)
                  n1672 = Index Array(array=w2772, index=w2768) -> (element=w2771:u8)
                  n1673 = Equal?(x=w2768, y=w2766) -> (x = y?=w2765:bool)
                  n1674 = Number To Decimal String(number=w2771) -> (decimal integer string=w2769:string)  [unwired: 1 in]
                  n1675 = Select(t="", s=w2765, f="\r") -> (s? t:f=w2762:string)
                  n1676 = Concatenate Strings(w2769, w2762) -> (w2770:string)
                }
                n1677 = local read "file path"() -> (w2734:path)
                n1678 = call <vilib>:"Read Characters From File.vi"("file path (dialog if empty)"=w2734) -> ("character string"=w2747:string)  [unwired: 5 in, 3 out]
                "string" <- w2747
                n1679 = flat-sequence {
                  tunnel: [w2750] -> _
                  frame #0 {
                    w2750 = ""
                    n1680 = local write "Password"(w2750) -> ()
                  }
                }
                n1681 = Concatenate Strings(w2738) -> (w2739:string)
                n1682 = Concatenate Strings(w2747) -> (w2746:string)
                n1683 = Concatenate Strings(w2749) -> (w2742:string)
                n1684 = Equal?(x=w2742, y=w2746) -> (x = y?=w2737:bool)
                n1685 = Equal?(x=w2742, y=w2739) -> (x = y?=w2743:bool)
                n1686 = Or(x=w2737, y=w2743) -> (x .or. y?=→"x = y?":bool)
              }
            }
          }
        }
        n1687 = local read "x = y?"() -> (w2718:bool)
        n1688 = And(x="EDIT", y=w2718) -> (x .and. y?=w2716:bool)
        n1689 = case shown="True" w2716 {
          tunnel: [u8 2 ("Disabled") u8 0 ("Disabled")] -> w2715
          tunnel: [w2922 TRUE ("Visible")] -> w2714
          frame False {
            w2922 = FALSE ("Visible")
            n1690 = local write "EDIT 2"(w2922) -> ()
          }
          frame True {
          }
        }
        n1691 = case shown="True" "SAVE" {
          frame False {
          }
          frame True {
            n1692 = stacked-sequence {
              seq-local: [w2777 _ _] -> [_ w2918 _]
              frame #0 {
                w2773 = 0.0 ("number")
                w2774 = 0.0 ("number")
                (unwired) i16 5 ("precision (6)")
                # "[CH1]    - FF\n[CH2]   - TEMPERATURE\n[CH3]    - Humidity\n[CH4]    - AIR TEMP\n[CH5]\\- Visa Uno\n[CH6] \\- Visa Due\n[CH7]  \\- file path\n[CH8]   - Displacement Gain\n[CHA]   - Stroke Gain\n[CHB]   - Stroke PID Gain\n[CHC]   -Language Selection\n[CHD]   -Power +\n[CHE]   -Power_\n[CHF]   -Heater\n[CHG]   -Humidity Wet\n[CHH]   -Humidity Dry\n[CHI]   -Integral Time"
                n1693 = local read "Language Selection"() -> (w2820:enum16{"English", "Russian"})
                n1694 = Path To String(path="File Path") -> (string=w2836:string)
                n1695 = Number To Fractional String(number=w2773, width (-)=i16 10 ("precision (6)"), precision (6)=i16 5) -> (F-format string=w2827:string)  [unwired: 1 in]
                n1696 = Number To Fractional String(number=w2820, width (-)=i16 10 ("precision (6)"), precision (6)=i16 5) -> (F-format string=w2816:string)  [unwired: 1 in]
                n1697 = Number To Fractional String(number=w2774, width (-)=i16 10 ("precision (6)"), precision (6)=i16 5) -> (F-format string=w2810:string)  [unwired: 1 in]
                n1698 = Number To Fractional String(number=w2774, width (-)=i16 10 ("precision (6)"), precision (6)=i16 5) -> (F-format string=w2807:string)  [unwired: 1 in]
                n1699 = Number To Fractional String(number=w2774, width (-)=i16 10 ("precision (6)"), precision (6)=i16 5) -> (F-format string=w2802:string)  [unwired: 1 in]
                n1700 = Number To Fractional String(number=w2774, width (-)=i16 10 ("precision (6)"), precision (6)=i16 5) -> (F-format string=w2799:string)  [unwired: 1 in]
                n1701 = Number To Fractional String(number=w2774, width (-)=i16 10 ("precision (6)"), precision (6)=i16 5) -> (F-format string=w2794:string)  [unwired: 1 in]
                n1702 = local read "Com Port 1"() -> (w2776:refnum<visa-resource-name>)
                n1703 = local read "Com Port 2"() -> (w2775:refnum<visa-resource-name>)
                n1704 = Concatenate Strings(w2836, "\\" ("string")) -> (w2835:string)
                n1705 = Number To Fractional String(number=w2773, width (-)=i16 10 ("precision (6)"), precision (6)=i16 5) -> (F-format string=w2868:string)  [unwired: 1 in]
                n1706 = Number To Fractional String(number=w2773, width (-)=i16 10 ("precision (6)"), precision (6)=i16 5) -> (F-format string=w2867:string)  [unwired: 1 in]
                n1707 = Number To Fractional String(number=w2773, width (-)=i16 10 ("precision (6)"), precision (6)=i16 5) -> (F-format string=w2861:string)  [unwired: 1 in]
                n1708 = Number To Fractional String(number=w2773, width (-)=i16 10 ("precision (6)"), precision (6)=i16 5) -> (F-format string=w2855:string)  [unwired: 1 in]
                n1709 = Number To Fractional String(number=w2773, width (-)=i16 10 ("precision (6)"), precision (6)=i16 5) -> (F-format string=w2828:string)  [unwired: 1 in]
                n1710 = Concatenate Strings("[CHA]" ("string"), w2827, "- Stroke Gain" ("string"), "\r") -> (w2821:string)
                n1711 = Concatenate Strings("[CHC]" ("string"), w2816, "-Language Selection" ("string"), "\r") -> (w2813:string)
                n1712 = Concatenate Strings("[CHD]" ("string"), w2810, "-Power +" ("string"), "\r") -> (w2792:string)
                n1713 = Concatenate Strings("[CHG]" ("string"), w2799, "-Humidity Wet" ("string"), "\r") -> (w2789:string)
                n1714 = Concatenate Strings("[CHH]" ("string"), w2794, "-Humidity Dry" ("string"), "\r") -> (w2788:string)
                n1715 = Concatenate Strings("[CH1]" ("string"), w2868, " - FF" ("string"), "\r") -> (w2866:string)
                n1716 = Concatenate Strings("[CH2]" ("string"), w2867, " - TEMPERATURE" ("string"), "\r") -> (w2865:string)
                n1717 = Concatenate Strings("[CH3]" ("string"), w2861, " - Humidity" ("string"), "\r") -> (w2858:string)
                n1718 = Concatenate Strings("[CH4]" ("string"), w2855, " - AIR TEMP" ("string"), "\r") -> (w2851:string)
                n1719 = Concatenate Strings("[CH5]" ("string"), w2776, "- Visa Uno" ("string"), "\r") -> (w2844:string)
                n1720 = Concatenate Strings("[CH6]" ("string"), w2775, "- Visa Due" ("string"), "\r") -> (w2839:string)
                n1721 = Concatenate Strings("[CH7]" ("string"), w2835, "- file path" ("string"), "\r") -> (w2838:string)
                n1722 = Concatenate Strings("[CH8]" ("string"), w2828, "- Displacement Gain" ("string"), "\r") -> (w2831:string)
                n1723 = Concatenate Strings("[CHE]" ("string"), w2807, "-Power_" ("string"), "\r") -> (w2791:string)
                n1724 = Concatenate Strings("[CHF]" ("string"), w2802, "-Heater" ("string"), "\r") -> (w2790:string)
                n1725 = Concatenate Strings(w2866, w2865, w2858, w2851, w2844, w2839, w2838, w2831, w2821, w2813, w2792, w2791, w2790, w2789, w2788) -> (w2777:string)
                "gain" <- w2777
              }
              frame #1 {
                w2879 = 0.0 ("number")
                n1726 = local read "Camera Port :"() -> (w2882:string)
                n1727 = local read "C3 :"() -> (w2890:refnum<visa-resource-name>)
                n1728 = local read "Com Port 3"() -> (w2891:refnum<visa-resource-name>)
                n1729 = Concatenate Strings("[CH8]" ("string"), w2882, "- Visa Camera" ("string"), "\r") -> (w2881:string)
                n1730 = Concatenate Strings("[CH7]" ("string"), w2890, "- Visa Humidity" ("string"), "\r") -> (w2886:string)
                n1731 = Number To Fractional String(number=w2879, width (-)=i16 10 ("precision (6)"), precision (6)=i16 5) -> (F-format string=w2906:string)  [unwired: 1 in]
                n1732 = Concatenate Strings("[CHL]" ("string"), w2891, "- Visa humid" ("string"), "\r") -> (w2894:string)
                n1733 = Number To Fractional String(number=w2879, width (-)=i16 10 ("precision (6)"), precision (6)=i16 5) -> (F-format string=w2913:string)  [unwired: 1 in]
                n1734 = Concatenate Strings("[CHK]" ("string"), w2906, "-TEMP INTERCEPT" ("string"), "\r") -> (w2902:string)
                n1735 = Concatenate Strings("[SNO]" ("string"), "" ("string"), "-" ("string"), "\r") -> (w2899:string)
                n1736 = Concatenate Strings("[CHJ]" ("string"), w2913, "-AIR TEMP INTERCEPT" ("string"), "\r") -> (w2903:string)
                n1737 = String To Path(string="C:\\LAB-IQ\\calibrate WO 2465.dcf") -> (path=w2892:path)
                n1738 = Concatenate Strings(w2918, w2903, w2902, w2899, w2894, w2886, w2881) -> (w2917:string)
                n1739 = call <vilib>:"Write Characters To File.vi"("append to file? (new file:F)"=FALSE, "character string"=w2917, "file path (dialog if empty)"=w2892) -> ()  [unwired: 2 in, 1 out]
              }
              frame #2 {
                n1740 = local write "Lan flag"(0.0 ("Lan flag")) -> ()
                n1741 = local write "conststatus"(0.0 ("rpm value : 2")) -> ()
                n1742 = local write "SAVE"(FALSE ("OK Button 14")) -> ()
              }
            }
          }
        }
        n1743 = property on="EDIT 2" class="Bool (strict)"("Visible"=w2714) -> ()  [unwired: 2 in, 2 out]
        n1744 = property on="SAVE" class="Bool (strict)"("Visible"=w2714) -> ()  [unwired: 2 in, 2 out]
        n1745 = property on="visa due" class="CmbBox"("Disabled"=w2715) -> ()  [unwired: 2 in, 2 out]
        n1746 = property on="File Path" class="Path"("Disabled"=w2715) -> ()  [unwired: 2 in, 2 out]
        n1747 = property on="Language Selection" class="Enum (strict)"("Visible"=w2714) -> ()  [unwired: 2 in, 2 out]
        n1748 = property on="SPEED OUT:" class="DigNum (strict)"("Disabled"=w2715) -> ()  [unwired: 2 in, 2 out]
      }
    }
    n1749 = local read "RUN"() -> (w2111:bool)
    n1750 = local read "RUN"() -> (w2109:bool)
    n1751 = disable-structure shown="Disabled" {
      disable-tunnel: [w2126 _] -> w2092
      disable-tunnel: [w2125 _] -> w2090
      frame Disabled {
        n1752 = local read "Temperature before test"() -> (w2119:dbl)
        n1753 = local read "Temperature after test"() -> (w2132:dbl)
        n1754 = case shown="True" "Save Results" {
          frame False {
          }
          frame True {
            w2148 = "\r"
            n1755 = local write "Save Results"(FALSE ("OK Button 5")) -> ()
            n1756 = local read "Temperature before test"() -> (w2186:dbl)
            n1757 = local read "Temperature after test"() -> (w2188:dbl)
            n1758 = local read "Humidity before test"() -> (w2185:dbl)
            n1759 = local read "Humidity after test"() -> (w2187:dbl)
            n1760 = local read "WS1.4"() -> (w2192:dbl)
            n1761 = local read "AVP"() -> (w2190:dbl)
            n1762 = Number To Fractional String(number=w2192, width (-)=i16 6, precision (6)=i16 1) -> (F-format string=w2152:string)  [unwired: 1 in]
            n1763 = local read "MWSD"() -> (w2189:dbl)
            n1764 = local read "String"() -> (w2181:string)
            n1765 = local read "FILE"() -> (w2184:string)
            n1766 = local read "HCF"() -> (w2191:dbl)
            n1767 = Number To Fractional String(number=w2185, width (-)=i16 6, precision (6)=i16 1) -> (F-format string=w2177:string)  [unwired: 1 in]
            n1768 = Number To Fractional String(number=w2186, width (-)=i16 6, precision (6)=i16 1) -> (F-format string=w2174:string)  [unwired: 1 in]
            n1769 = Number To Fractional String(number=w2187, width (-)=i16 6, precision (6)=i16 1) -> (F-format string=w2170:string)  [unwired: 1 in]
            n1770 = Number To Fractional String(number=w2188, width (-)=i16 6, precision (6)=i16 1) -> (F-format string=w2166:string)  [unwired: 1 in]
            n1771 = Number To Fractional String(number=w2190, width (-)=i16 6, precision (6)=i16 3) -> (F-format string=w2159:string)  [unwired: 1 in]
            n1772 = Concatenate Strings(w2181, w2184) -> (w2203:string)
            n1773 = Number To Fractional String(number=w2189, width (-)=i16 6, precision (6)=i16 1) -> (F-format string=w2163:string)  [unwired: 1 in]
            n1774 = Number To Fractional String(number=w2191, width (-)=i16 6, precision (6)=i16 2) -> (F-format string=w2157:string)  [unwired: 1 in]
            n1775 = Concatenate Strings("(" ("string"), w2152, ")Microns" ("string")) -> (w2151:string)
            n1776 = local read "REMARKS"() -> (w2183:string)
            "REMARKS 2" <- w2183
            n1777 = Concatenate Strings("(" ("string"), w2177, " ) % RH," ("string")) -> (w2178:string)
            n1778 = Concatenate Strings(w2157, ")" ("string")) -> (w2155:string)
            n1779 = Concatenate Strings("(" ("string"), w2174, ")  Deg C ," ("string")) -> (w2173:string)
            n1780 = Concatenate Strings("(" ("string"), w2170, " ) % RH," ("string")) -> (w2169:string)
            n1781 = Concatenate Strings("(" ("string"), w2166, ")  Deg C ," ("string")) -> (w2165:string)
            n1782 = Concatenate Strings("(" ("string"), w2163, ")  Microns," ("string")) -> (w2162:string)
            n1783 = Concatenate Strings("(" ("string"), w2159, ")  kPa," ("string")) -> (w2149:string)
            n1784 = Concatenate Strings(w2203, ".dwm" ("Substring")) -> (w2201:string)
            n1785 = String To Path(string=w2201) -> (path=w2200:path)
            n1786 = Concatenate Strings(w2183, w2148, " Humidity before test= " ("Substring"), w2178, w2148, " Temperature before test = " ("Substring"), w2173, w2148, " Humidity after test= " ("Substring"), w2169, w2148, "Temperature after test = " ("Substring"), w2165, w2148, "MSD = " ("Substring"), w2162, w2148, "  AVP = " ("Substring"), w2149, w2148, "  HCF                     =( " ("Substring"), w2155, w2148, " WS1.4                  = " ("Substring"), w2151, w2148) -> (w2147:string)
            "data" <- w2147
            n1787 = call <vilib>:"Write Characters To File.vi"("append to file? (new file:F)"=FALSE, "character string"=w2147, "file path (dialog if empty)"=w2200) -> ()  [unwired: 2 in, 1 out]
            n1788 = Match Pattern(string=w2147, regular expression="!") -> (after substring=→"export":string)  [unwired: 1 in, 3 out]
          }
        }
        n1789 = Add(x=231.864, y=w2119) -> (x+y=w2116:dbl)
        n1790 = Add(x=231.864, y=w2132) -> (x+y=w2129:dbl)
        n1791 = Divide(x=1705.984, y=w2116) -> (x/y=w2117:dbl)
        n1792 = Divide(x=1705.984, y=w2129) -> (x/y=w2130:dbl)
        n1793 = local read "Humidity before test"() -> (w2121:dbl)
        n1794 = local read "Humidity after test"() -> (w2134:dbl)
        n1795 = Subtract(x=8.017352 ("y"), y=w2117) -> (x-y=w2143:dbl)
        n1796 = Subtract(x=8.017352 ("y"), y=w2130) -> (x-y=w2137:dbl)
        n1797 = expression code="10**y"(w2143) -> (w2123:dbl)
        n1798 = expression code="10**y"(w2137) -> (w2136:dbl)
        n1799 = Multiply(x=w2121, y=w2123) -> (x*y=w2122:dbl)
        n1800 = Multiply(x=w2134, y=w2136) -> (x*y=w2135:dbl)
        n1801 = Divide(x=w2122, y=750.0) -> (x/y=w2138:dbl)
        n1802 = Divide(x=w2135, y=750.0) -> (x/y=w2139:dbl)
        n1803 = Add(x=w2138, y=w2139) -> (x+y=w2140:dbl)
        n1804 = Divide(x=w2140, y=2.0) -> (x/y=w2142:dbl)
        n1805 = local write "AVP"(w2142) -> ()
        n1806 = Subtract(x=1.4, y=w2142) -> (x-y=w2125:dbl)
        n1807 = local read "HCF"() -> (w2126:dbl)
      }
      frame Enabled {
      }
    }
    n1808 = case shown="True" "EDIT 3" {
      frame False {
      }
      frame True {
        n1809 = local write "EDIT 3"(FALSE ("EDIT 3")) -> ()
        n1810 = local write "Main Tab"(T2."About" ("Main Tab")) -> ()
      }
    }
    n1811 = case shown="False" w2111 {
      frame False {
        n1812 = local read "stopT"() -> (w2929:bool)
        n1813 = case shown="True" w2929 {
          frame False {
          }
          frame True {
            n1814 = local write "stopT"(FALSE) -> ()
          }
        }
      }
      frame True {
        "stopT" <- TRUE
      }
    }
    n1815 = case shown="False" w2109 {
      frame False {
      }
      frame True {
      }
    }
    n1816 = case shown="True" w2099 {
      frame False {
        n1817 = property on="Password 2" class="Str"("Visible"=FALSE) -> ()  [unwired: 2 in, 2 out]
        n1818 = local write "Password 2"("" ("Password")) -> ()
      }
      frame True {
        n1819 = property on="Password 2" class="Str"("Visible"=TRUE) -> ()  [unwired: 2 in, 2 out]
        n1820 = Equal?(x="Password 2", y="HFRR1234") -> (x = y?=w2231:bool)
        n1821 = case shown="True" w2231 {
          tunnel: "Password 2" -> [w2234 _]
          frame False {
            n1822 = String Length(string=w2234) -> (length=w2235:i32)
            n1823 = Greater Than 0?(x=w2235) -> (x > 0?=w2233:bool)
            n1824 = case shown="False" w2233 {
              frame False {
                n1825 = property on="Password 2" class="Str"("Caption.Text"="Password (Advance Setting)") -> ()  [unwired: 2 in, 2 out]
              }
              frame True {
                n1826 = property on="Password 2" class="Str"("Caption.Text"="Incorrect Password!") -> ()  [unwired: 2 in, 2 out]
              }
            }
          }
          frame True {
            n1827 = local write "EDIT 2"(FALSE ("EDIT 2")) -> ()
            n1828 = local write "Password 2"("" ("Password")) -> ()
            n1829 = local write "Main Tab"(T2."Advance" ("Main Tab")) -> ()
            n1830 = local write "Main Dashboard Buttons"(T1."Advance" ("Main Dashboard Buttons")) -> ()
          }
        }
      }
    }
    n1831 = case shown="True" "Prog Uno" {
      frame False {
      }
      frame True {
        n1832 = stacked-sequence {
          frame #0 {
            n1833 = Delete(path (use dialog)=path "C:/LAB-IQ-NXT/UNOCOMPILE.bat" ("working directory")) -> ()  [unwired: 4 in, 3 out]
          }
          frame #1 {
            n1834 = local read "Com Port 1"() -> (w2696:refnum<visa-resource-name>)
            n1835 = Concatenate Strings("cmd.exe /c \"mode " ("command line"), w2696, ":1200,n,8,1\"\n" ("command line")) -> (w2701:string)
            n1836 = Concatenate Strings(w2701, "CD\\\nCD WinDucom\navrdude -C avrdude.conf -v -patmega328p -carduino -P" ("command line"), w2696, " -b115200 -D -Uflash:w:UNO_V20.hex:i\n" ("command line"), "\r") -> (w2703:string)
            "STR" <- w2703
            n1837 = call <vilib>:"Write Characters To File.vi"("append to file? (new file:F)"=FALSE, "character string"=w2703, "file path (dialog if empty)"=path "C:/LAB-IQ/UNOCOMPILE.bat" ("working directory")) -> ()  [unwired: 2 in, 1 out]
          }
          frame #2 {
            n1838 = disable-structure shown="Disabled" {
              frame Disabled {
                w2707 = "cmd.exe  /c \"C:\\LAB-IQ-NXT\\UNOCOMPILE.bat\"" ("string")
                n1839 = local write "Prog Uno"(FALSE ("run minimized? (F)")) -> ()
                n1840 = call <vilib>:"System Exec.vi"("expected output size  (4096)"=u32 65535, "run minimized? (F)"=FALSE, "wait until completion? (T)"=TRUE ("run minimized? (F)"), "working directory"=path "C:/LAB-IQ-NXT", "standard input"=w2707, "command line"=w2707) -> ("error out"=w2706:errorcluster, "standard output"=→"String 42":string)  [unwired: 2 in, 2 out]
                "error out 3" <- w2706
                n1841 = flat-sequence {
                  tunnel: w2706 -> [_]
                  frame #0 {
                  }
                }
              }
              frame Enabled {
              }
            }
          }
        }
      }
    }
    n1842 = case shown="\"ISO 12156\"" "TEST STANDARD" {
      tunnel: [2.0 ("Set Temp") 0.0 ("Set Temp") 2.0 ("Set Temp") 0.0 ("Set Temp")] -> w2100
      frame "ASTM D6079", Default {
        w2653 = 50.0 ("Hz")
        w2654 = 53.0 ("Set Rh")
        w2656 = 1.0 ("Set Strk")
        w2655 = 60.0 ("Set Temp")
        # "astm hide"
        n1843 = local write "NORMAL LOAD"(200.0 ("NORMAL LOAD")) -> ()
        n1844 = local write "Set Strk"(w2656) -> ()
        n1845 = local write "Set Hz"(w2653) -> ()
        n1846 = local write "Set Temp"(w2655) -> ()
        n1847 = local write "Set Rh"(w2654) -> ()
        n1848 = local write "test time"(75.0 ("test time")) -> ()
        n1849 = local write "Set Stroke:"(w2656) -> ()
        n1850 = local write "Set Humidity:"(w2654) -> ()
        n1851 = local write "Set Frequency:"(w2653) -> ()
        n1852 = local write "Set Temperature:"(w2655) -> ()
        "Test Standard" <- "ASTM D6079" ("Test Standard 2")
      }
      frame "ISO 12156" {
        n1853 = local write "Set Strk"(1.0 ("Set Strk")) -> ()
        n1854 = local write "NORMAL LOAD"(200.0 ("NORMAL LOAD")) -> ()
        n1855 = local write "Set Temp"(60.0 ("Set Temp")) -> ()
        n1856 = local write "test time"(75.0 ("test time")) -> ()
        n1857 = local write "Set Hz"(50.0 ("Hz")) -> ()
        n1858 = local write "Set Rh"(53.0 ("Set Rh")) -> ()
      }
      frame "CEC F-096-A-06" {
        n1859 = local write "Set Strk"(1.0 ("Set Strk")) -> ()
        n1860 = local write "NORMAL LOAD"(200.0 ("NORMAL LOAD")) -> ()
        n1861 = local write "Set Temp"(60.0 ("Set Temp")) -> ()
        n1862 = local write "test time"(75.0 ("test time")) -> ()
        n1863 = local write "Set Hz"(50.0 ("Hz")) -> ()
        n1864 = local write "Set Rh"(53.0 ("Set Rh")) -> ()
      }
      frame "Custom" {
      }
    }
    n1865 = case shown="True" "Prog Due" {
      frame False {
      }
      frame True {
        n1866 = stacked-sequence {
          frame #0 {
            n1867 = Delete(path (use dialog)=path "C:/LAB-IQ/DUECOMPILE.bat" ("working directory")) -> ()  [unwired: 4 in, 3 out]
          }
          frame #1 {
            n1868 = disable-structure shown="Disabled" {
              frame Disabled {
                n1869 = local read "visa due"() -> (w2678:string)
                n1870 = Concatenate Strings("cmd.exe /c \"mode " ("command line"), w2678, ":1200,n,8,1\"\n" ("command line")) -> (w2683:string)
                n1871 = Concatenate Strings(w2683, "CD\\\nCD WinDucom\nTIMEOUT 1\n bossac.exe -i -d --port=" ("command line"), w2678, " -U false -e -w -v -b DUE.bin -R\n" ("command line"), "\r") -> (w2685:string)
                "concatenated string 2" <- w2685
                n1872 = call <vilib>:"Write Characters To File.vi"("append to file? (new file:F)"=FALSE, "character string"=w2685, "file path (dialog if empty)"=path "C:/LAB-IQ-NXT/DUECOMPILE.bat" ("working directory")) -> ()  [unwired: 2 in, 1 out]
              }
              frame Enabled {
              }
            }
          }
          frame #2 {
            # "C:\\LAB-IQ-NXT\\DUECOMPILE.bat"
            n1873 = disable-structure shown="Disabled" {
              frame Disabled {
                w2690 = "cmd.exe  /c \"C:\\LAB-IQ-NXT\\DUECOMPILE.bat\"" ("string")
                n1874 = call <vilib>:"System Exec.vi"("expected output size  (4096)"=u32 65535, "run minimized? (F)"=FALSE, "wait until completion? (T)"=TRUE ("run minimized? (F)"), "working directory"=path "C:/LAB-IQ-NXT", "standard input"=w2690, "command line"=w2690) -> ("error out"=w2689:errorcluster, "standard output"=→"String 44":string)  [unwired: 2 in, 2 out]
                "error out 4" <- w2689
                n1875 = flat-sequence {
                  tunnel: w2689 -> [_]
                  frame #0 {
                  }
                }
              }
              frame Enabled {
              }
            }
            n1876 = local write "Prog Due"(FALSE ("Prog Due")) -> ()
          }
        }
      }
    }
    n1877 = Or(x=w2097, y=w2095) -> (x .or. y?=w2096:bool)
    n1878 = case shown="\"About\"" w2094 {
      tunnel: [T25."Acquire" ("Main Tab") T25."Compare Files" ("Main Tab") T25."About" ("Main Tab")] -> w2107
      frame "Acquire", Default {
      }
      frame "Compare Files" {
      }
      frame "About" {
      }
    }
    n1879 = Or(x=w2101, y="OPEN") -> (x .or. y?=w2102:bool)
    n1880 = case shown="True" w2102 {
      tunnel: w2101 -> [_ w2242]
      frame False {
      }
      frame True {
        n1881 = stacked-sequence {
          tunnel: w2242 -> [_ w2309 _ _]
          frame #0 {
            w2258 = "  " ("String 6")
            n1882 = local write "OPEN"(FALSE ("open")) -> ()
            n1883 = local read "string1 2"() -> (w2246:string)
            n1884 = local read "string1 3"() -> (w2245:string)
            n1885 = local read "string1 4"() -> (w2244:string)
            n1886 = property on="OPEN" class="Bool (strict)"("Visible"=FALSE) -> ()  [unwired: 2 in, 2 out]
            n1887 = local write "String 6"(w2258) -> ()
            n1888 = local write "String 7"(w2258) -> ()
            n1889 = local write "String 8"(w2258) -> ()
            n1890 = local write "String 12"(w2258) -> ()
            n1891 = local read "OK Button 16"() -> (w2243:bool)
            n1892 = String To Path(string=w2246) -> (path=w2254:path)
            n1893 = String To Path(string=w2245) -> (path=w2253:path)
            n1894 = String To Path(string=w2244) -> (path=w2252:path)
            n1895 = case shown="True" w2243 {
              tunnel: [w2259 w2260] -> w2247
              frame False {
                n1896 = local read "string1"() -> (w2259:string)
              }
              frame True {
                n1897 = local read "String Indicator 4"() -> (w2260:string)
              }
            }
            n1898 = Open/Create/Replace File "Open File"(file path (use dialog)=w2254) -> (refnum out=w2250:refnum<file>)  [unwired: 5 in, 2 out]
            n1899 = Open/Create/Replace File "Open File"(file path (use dialog)=w2253) -> (refnum out=w2249:refnum<file>)  [unwired: 5 in, 2 out]
            n1900 = Open/Create/Replace File "Open File"(file path (use dialog)=w2252) -> (refnum out=w2248:refnum<file>)  [unwired: 5 in, 2 out]
            n1901 = while {
              tunnel: w2250 -> [w2272]
              i -> [w2268]
              stop <- w2267 continue-if-true
              (unwired) TRUE ("line mode (F)")
              n1902 = Read from Text File "Read File"(file (use dialog)=w2272) -> (text=w2269:string)  [unwired: 3 in, 3 out]
              n1903 = local write "Numeric 11"(w2268) -> ()
              n1904 = String Length(string=w2269) -> (length=w2271:i32)
              n1905 = Greater?(x=w2271, y=1) -> (0:w2267:bool)
            }
            n1906 = while {
              tunnel: w2249 -> [w2278]
              i -> [w2274]
              stop <- w2273 continue-if-true
              (unwired) TRUE ("line mode (F)")
              n1907 = Read from Text File "Read File"(file (use dialog)=w2278) -> (text=w2275:string)  [unwired: 3 in, 3 out]
